vi "Fetch Waveform.vi"   [LabVIEW 2009, in "Tektronix DPO MSO 2000 4000 Series.lvlib"]
doc: "The polymorphic VI returns waveform data that an oscilloscope acquired for a channel you specify. You select to use the <B>tkdpo4k Fetch Waveform (1DI16 (unscaled))</B> VI if you choose to get raw waveform data. You select to use the <B>todpo4k Fetch Waveform (Waveform Data Type)</B> VI if you choose to get scaled waveform data."
uses:
  <instrlib>/Tektronix DPO MSO 2000 4000 Series/Tektronix DPO MSO 2000 4000 Series.lvlib
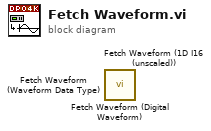
[diagram p0: block diagram]
diagram:
  n1 = call <instrlib>:"Fetch Waveform (Digital Waveform).vi"() -> ()  [unwired: 9 in, 3 out]
  n2 = call <instrlib>:"Fetch Waveform (1D I16 (unscaled)).vi"() -> ()  [unwired: 7 in, 5 out]
  n3 = call <instrlib>:"Fetch Waveform (Waveform Data Type).vi"() -> ()  [unwired: 9 in, 3 out]
